vi "lvEtherbone.socket_open.vi"(0 "port":string, 5 "error in (no error)":errorcluster) -> (13 "eb_status":T1 items=["EB_SUCCESS"=1, "EB_OK"=0, "EB_FAIL"=-1, "EB_ADDRESS"=-2, "EB_WIDTH"=-3, "EB_OVERFLOW"=-4, "EB_ENDIAN"=-5, "EB_BUSY"=-6, "EB_TIMEOUT"=-7, "EB_OOM"=-8, "EB_ABI"=-9, "EB_SEGFAULT"=-10], 14 "eb_socket_ID":i32, 19 "error out":errorcluster)   [LabVIEW 2012, in "lvEtherbone.lvlib"]
doc: "/* Open an Etherbone socket for communicating with remote devices.\n * Open sockets must be hooked into an event loop; see eb_socket_{run,check}.\n * \n * The abi_code must be EB_ABI_CODE. This confirms library compatability.\n * The port parameter is optional; 0 lets the operating system choose.\n * Supported_widths list bus widths acceptable to the local Wishbone bus.\n * EB_ADDR32|EB_ADDR8|EB_DATAX means 8/32-bit addrs and 8/16/32/64-bit data.\n * Devices opened by this socket only negotiate a subset of these widths.\n * Virtual slaves attached to the socket never see a width excluded here.\n *\n * Return codes:\n * OK - successfully open the socket port\n * FAIL - operating system forbids access\n * BUSY - specified port is in use (only possible if port != 0)\n * WIDTH - supported_widths were invalid\n * OOM - out of memory\n * ABI - library is not compatible with application\n */\nEB_PUBLIC\neb_status_t eb_socket_open(uint16_t abi_code,\n const char* port, \n eb_width_t supported_widths,\n eb_socket_t* result);"
uses:
  lvEtherbone.lvlib
  lvEtherbone.lveb_status_t.ctl
  libetherbone.so
panel:
  in  "eb_status_t":T1 items=["EB_SUCCESS"=1, "EB_OK"=0, "EB_FAIL"=-1, "EB_ADDRESS"=-2, "EB_WIDTH"=-3, "EB_OVERFLOW"=-4, "EB_ENDIAN"=-5, "EB_BUSY"=-6, "EB_TIMEOUT"=-7, "EB_OOM"=-8, "EB_ABI"=-9, "EB_SEGFAULT"=-10]
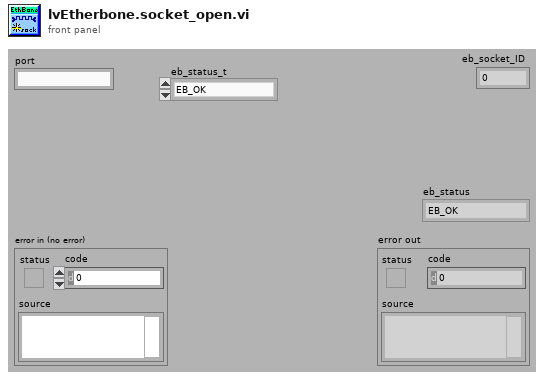
[diagram p1: front panel]
types:
  T1 = typedef "lvEtherbone.lvlib/lvEtherbone.lveb_status_t.ctl" = i32
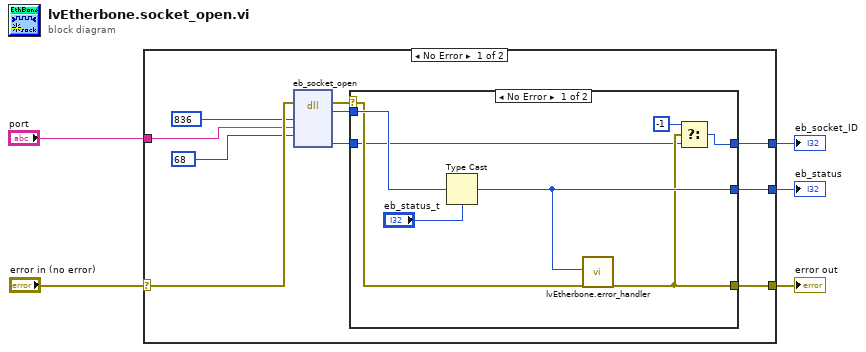
[diagram p0: block diagram]
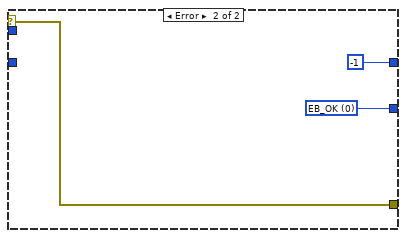
[diagram p2: hidden frame]
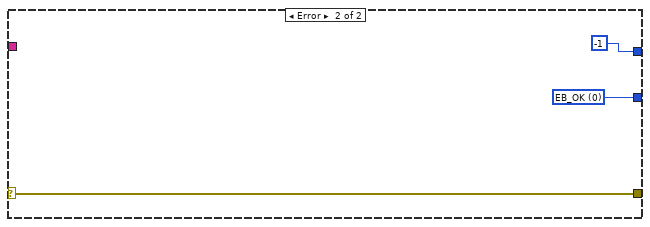
[diagram p3: hidden frame]
diagram:
  n1 = case shown="No Error" "error in (no error)" {
    selector: "error in (no error)" -> [w15 w29]
    tunnel: [w12 w29] -> w4
    tunnel: [w13 w28] -> w3
    tunnel: [w11 -1 ("eb_socket_ID")] -> w2
    tunnel: "port" -> [w6 _]
    frame No Error {
      n2 = dll-call lib="libetherbone.so" fn="eb_socket_open"(error in=w15, "abi_code"=u16 836, "port"=w6, "supported_widths"=u8 68 ("abi_code")) -> (error out=w10:errorcluster, "eb_status"=w14:i32, "eb_socket_t"=w7:u16)  [unwired: 6 in, 1 out]
      n3 = case shown="No Error" w10 {
        selector: w10 -> [w20 w26]
        tunnel: w14 -> [w23 _]
        tunnel: [w21 w24] -> w13
        tunnel: [w19 w26] -> w12
        tunnel: w7 -> [w18 _]
        tunnel: [w17 -1 ("eb_socket_ID")] -> w11
        frame No Error {
          n4 = Type Cast(type="eb_status_t", x=w23) -> (*(type *) &x=w21:T1)
          n5 = call "lvEtherbone.error_handler.vi"("eb_status"=w21, "error in"=w20) -> ("error out"=w19:errorcluster)  [unwired: 17 in]
          n6 = Select(t=-1, s=w19, f=w18) -> (s? t:f=w17:i32)
        }
        frame Error {
          w24 = T1 0 items=["EB_SUCCESS"=1, "EB_OK"=0, "EB_FAIL"=-1, "EB_ADDRESS"=-2, "EB_WIDTH"=-3, "EB_OVERFLOW"=-4, "EB_ENDIAN"=-5, "EB_BUSY"=-6, "EB_TIMEOUT"=-7, "EB_OOM"=-8, "EB_ABI"=-9, "EB_SEGFAULT"=-10] ("eb_status_t")
        }
      }
    }
    frame Error {
      w28 = T1 0 items=["EB_SUCCESS"=1, "EB_OK"=0, "EB_FAIL"=-1, "EB_ADDRESS"=-2, "EB_WIDTH"=-3, "EB_OVERFLOW"=-4, "EB_ENDIAN"=-5, "EB_BUSY"=-6, "EB_TIMEOUT"=-7, "EB_OOM"=-8, "EB_ABI"=-9, "EB_SEGFAULT"=-10] ("eb_status_t")
    }
  }
  "error out" <- w4
  "eb_status" <- w3
  "eb_socket_ID" <- w2
